vi "Attenuator Append Group Data Fields.vi"(10 "Attenuator Results":T1={"Measurement Cycles"=0, "Attenuator Test Parameters"={"Stimulus"={"ATT Stimulus"={"Normalize"=TRUE, "Value (dB)"=0.0}, "VNA Stimulus"={"Use Instrument Settings"=FALSE, "Blank Frequencies"=FALSE, "Sweep Type"=enum."Linear", "Sweep"={"Fstart"=500.0, "Fstop"=1500.0, "Units"=enum."MHz", "Points"=201}, "Power (dBm)"=999.0, "IFBW (Hz)"=-1.0, "Sweep Time (s)"=-1.0, "Calibration"={"State"=FALSE, "String"=""}}}, "Measurement"={"Step (dB)"=enum."0.25", "Start (dB)"=0.0, "Stop (dB)"=31.75}, "Limit"={"Maximum Error"=0.3}, "Normalization"={"Normalized?"=FALSE, "Normalization Values (dB)"=[]}}, "Measurement Values"={"# of Steps"=0, "Attenuation Variance"=[], "Frequency Sweeps"=[], "Peak Variance (dB)"=0.0, "Monotonic?"=FALSE}, "Pass?"=FALSE, "Instruments to Use"={"ATT Instrument Record"={"ixInstrument"=0, "sxInstrumentId"="", "sDriverId"="", "sDriverType"="", "sSerialNumber"="", "tLastCalibration"=timestamp(0 s since 1904-01-01), "tCalibrationDue"=timestamp(0 s since 1904-01-01), "sConfiguration"=""}, "VNA Instrument Record"={"ixInstrument"=0, "sxInstrumentId"="", "sDriverId"="", "sDriverType"="", "sSerialNumber"="", "tLastCalibration"=timestamp(0 s since 1904-01-01), "tCalibrationDue"=timestamp(0 s since 1904-01-01), "sConfiguration"=""}}} {"Attenuator Test Parameters"."Stimulus"."VNA Stimulus"."Sweep Time (s)" format="%.3g"}, 11 "Fields In":T13[](array[typedef])) -> (3 "Fields Out":T13[](array[typedef]))   [LabVIEW 2011]
uses:
  server/database/Fields/Field Record.ctl
  server/database/Fields/Field DataTypes.ctl
  server/database/Fields/Field NextItem.ctl
  TypeDefs/Attenuator Results.ctl
  TypeDefs/Attenuator Test Parameters.ctl
  TypeDefs/Attenuator Stimulus Parameters.ctl
  TypeDefs/Attenuator ATT Stimulus.ctl
  TypeDefs/Attenuator VNA Stimulus.ctl
  S Parameter/TypeDefs/SP Frequency Units.ctl
  TypeDefs/Attenuator VNA Calibration State.ctl
  TypeDefs/Attenuator Measurement Cluster.ctl
  TypeDefs/Attenuator Limit.ctl
  TypeDefs/Attenuator Calibration State.ctl
  TypeDefs/Attenuator Measurement Values.ctl
  server/database/Stations/Instruments/Instrument Record.ctl
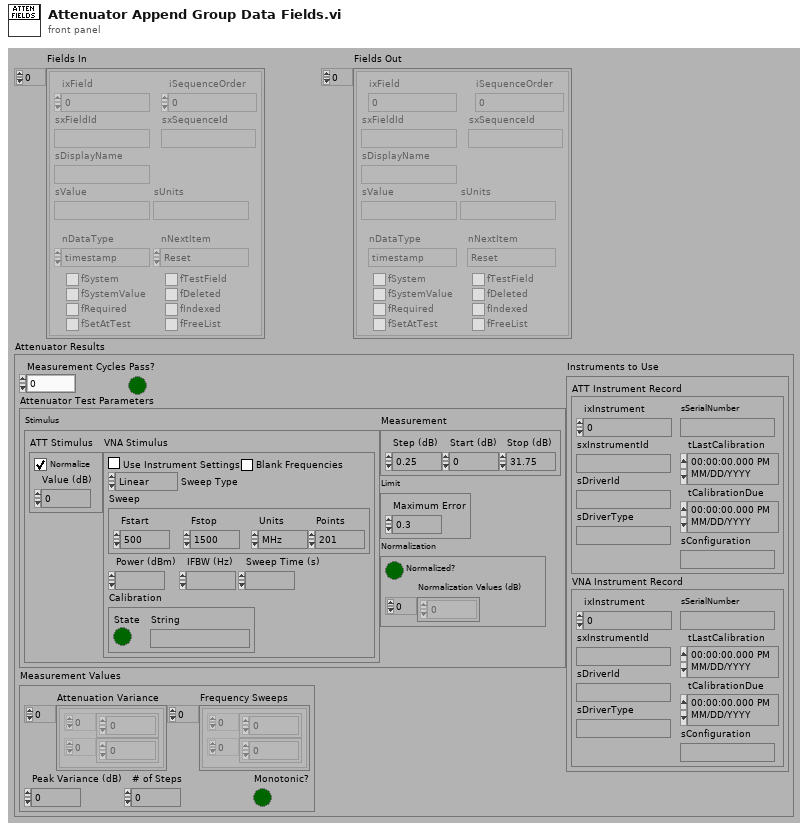
[diagram p1: front panel]
types:
  T1 = typedef "Attenuator Results.ctl" = cluster{"Measurement Cycles":i32, "Attenuator Test Parameters":T2, "Measurement Values":T11, "Pass?":bool, "Instruments to Use":cluster{"ATT Instrument Record":T12, "VNA Instrument Record":T12}}
  T2 = typedef "Attenuator Test Parameters.ctl" = cluster{"Stimulus":T3, "Measurement":T8, "Limit":T9, "Normalization":T10}
  T3 = typedef "Attenuator Stimulus Parameters.ctl" = cluster{"ATT Stimulus":T4, "VNA Stimulus":T5}
  T4 = typedef "Attenuator ATT Stimulus.ctl" = cluster{"Normalize":bool, "Value (dB)":dbl}
  T5 = typedef "Attenuator VNA Stimulus.ctl" = cluster{"Use Instrument Settings":bool, "Blank Frequencies":bool, "Sweep Type":enum32{"Linear", "Logarithmic", "List", "Power", "CW"}, "Sweep":cluster{"Fstart":dbl, "Fstop":dbl, "Units":T6, "Points":i32}, "Power (dBm)":dbl, "IFBW (Hz)":dbl, "Sweep Time (s)":dbl, "Calibration":T7}
  T6 = typedef "SP Frequency Units.ctl" = enum16{"Hz", "kHz", "MHz", "GHz", "Points"}
  T7 = typedef "Attenuator VNA Calibration State.ctl" = cluster{"State":bool, "String":string}
  T8 = typedef "Attenuator Measurement Cluster.ctl" = cluster{"Step (dB)":enum16{"0.25", "0.50", "1.00"}, "Start (dB)":dbl, "Stop (dB)":dbl}
  T9 = typedef "Attenuator Limit.ctl" = cluster{"Maximum Error":dbl}
  T10 = typedef "Attenuator Calibration State.ctl" = cluster{"Normalized?":bool, "Normalization Values (dB)":dbl[]}
  T11 = typedef "Attenuator Measurement Values.ctl" = cluster{"# of Steps":i32, "Attenuation Variance":cluster{"X":dbl[], "Y":dbl[]}[], "Frequency Sweeps":cluster{"X":dbl[], "Y":dbl[]}[], "Peak Variance (dB)":dbl, "Monotonic?":bool}
  T12 = typedef "Instrument Record.ctl" = cluster{"ixInstrument":i32, "sxInstrumentId":string, "sDriverId":string, "sDriverType":string, "sSerialNumber":string, "tLastCalibration":timestamp, "tCalibrationDue":timestamp, "sConfiguration":string}
  T13 = typedef "Field Record.ctl" = cluster{"ixField":i32, "iSequenceOrder":i32, "sxFieldId":string, "sxSequenceId":string, "sDisplayName":string, "sValue":string, "sUnits":string, "nDataType":T14, "nNextItem":T15, "fSystem":bool, "fSystemValue":bool, "fRequired":bool, "fSetAtTest":bool, "fTestField":bool, "fDeleted":bool, "fIndexed":bool, "fFreeList":bool}
  T14 = typedef "Field DataTypes.ctl" = enum32{"text", "numeric", "list", "timestamp", "boolean"}
  T15 = typedef "Field NextItem.ctl" = enum32{"Reset", "Retain", "Auto-Increment"}
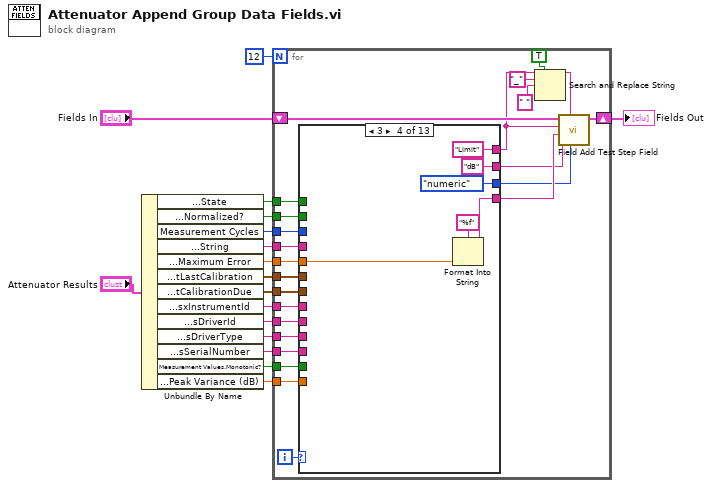
[diagram p0: block diagram]
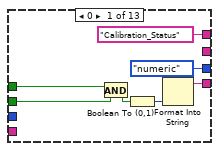
[diagram p2: hidden frame]
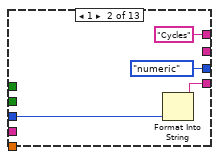
[diagram p3: hidden frame]
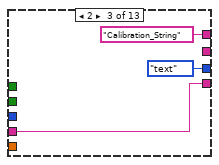
[diagram p4: hidden frame]
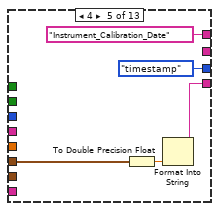
[diagram p5: hidden frame]
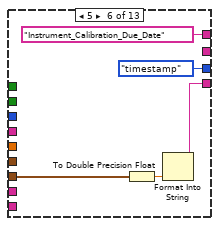
[diagram p6: hidden frame]
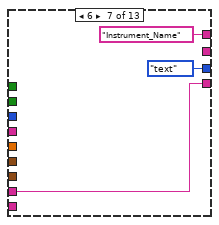
[diagram p7: hidden frame]
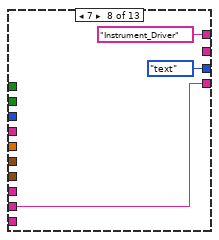
[diagram p8: hidden frame]
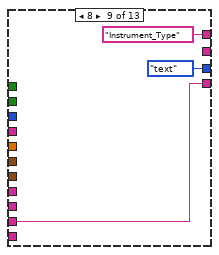
[diagram p9: hidden frame]
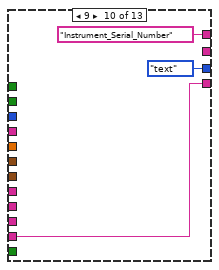
[diagram p10: hidden frame]
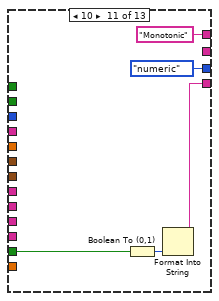
[diagram p11: hidden frame]
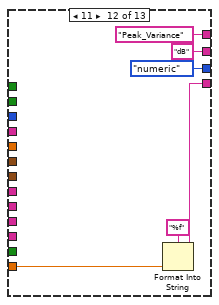
[diagram p12: hidden frame]
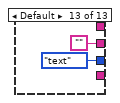
[diagram p13: hidden frame]
diagram:
  n1 = Unbundle By Name("Attenuator Results") -> ("Attenuator Test Parameters.Stimulus.VNA Stimulus.Calibration.State"=w3:bool, "Attenuator Test Parameters.Normalization.Normalized?"=w13:bool, "Measurement Cycles"=w12:i32, "Attenuator Test Parameters.Stimulus.VNA Stimulus.Calibration.String"=w11:string, "Attenuator Test Parameters.Limit.Maximum Error"=w10:dbl, "Instruments to Use.VNA Instrument Record.tLastCalibration"=w9:timestamp, "Instruments to Use.VNA Instrument Record.tCalibrationDue"=w4:timestamp, "Instruments to Use.VNA Instrument Record.sxInstrumentId"=w8:string, "Instruments to Use.ATT Instrument Record.sDriverId"=w7:string, "Instruments to Use.ATT Instrument Record.sDriverType"=w6:string, "Instruments to Use.ATT Instrument Record.sSerialNumber"=w5:string, "Measurement Values.Monotonic?"=w2:bool, "Measurement Values.Peak Variance (dB)"=w1:dbl)
  n2 = for {
    N: 12 -> [_]
    tunnel: w10 -> [w40]
    tunnel: w11 -> [w39]
    tunnel: w12 -> [w38]
    tunnel: w13 -> [w37]
    shift-right: [w35] -> w16
    shift-left: "Fields In" -> [w36]
    tunnel: w9 -> [w31]
    tunnel: w8 -> [w30]
    tunnel: w7 -> [w29]
    tunnel: w6 -> [w28]
    tunnel: w5 -> [w27]
    tunnel: w4 -> [w21]
    tunnel: w3 -> [w20]
    tunnel: w2 -> [w19]
    tunnel: w1 -> [w18]
    i -> [w41]
    n3 = case shown="3" w41 {
      tunnel: w40 -> [_ _ _ w58 _ _ _ _ _ _ _ _ _]
      tunnel: w39 -> [_ _ w53 _ _ _ _ _ _ _ _ _ _]
      tunnel: w38 -> [_ w50 _ _ _ _ _ _ _ _ _ _ _]
      tunnel: w37 -> [w44 _ _ _ _ _ _ _ _ _ _ _ _]
      tunnel: ["Calibration_Status" ("Field_ID") "Cycles" ("Field_ID") "Calibration_String" ("Field_ID") "Limit" ("Field_ID") "Instrument_Calibration_Date" ("Field_ID") "Instrument_Calibration_Due_Date" ("Field_ID") "Instrument_Name" ("Field_ID") "Instrument_Driver" ("Field_ID") "Instrument_Type" ("Field_ID") "Instrument_Serial_Number" ("Field_ID") "Monotonic" ("Field_ID") "Peak_Variance" ("Field_ID") _] -> w23
      tunnel: [Field_DataTypes."numeric" ("Data Type") Field_DataTypes."numeric" ("Data Type") Field_DataTypes."text" ("Data Type") Field_DataTypes."numeric" ("Data Type") Field_DataTypes."timestamp" ("Data Type") Field_DataTypes."timestamp" ("Data Type") Field_DataTypes."text" ("Data Type") Field_DataTypes."text" ("Data Type") Field_DataTypes."text" ("Data Type") Field_DataTypes."text" ("Data Type") Field_DataTypes."numeric" ("Data Type") Field_DataTypes."numeric" ("Data Type") Field_DataTypes."text" ("Data Type")] -> w33
      tunnel: [w47 w51 w53 w59 w63 w68 w72 w75 w78 w81 w84 w92 _] -> w34
      tunnel: [_ _ _ "dB" _ _ _ _ _ _ _ "dB" ""] -> w32
      tunnel: w31 -> [_ _ _ _ w62 _ _ _ _ _ _ _ _]
      tunnel: w30 -> [_ _ _ _ _ _ w72 _ _ _ _ _ _]
      tunnel: w29 -> [_ _ _ _ _ _ _ w75 _ _ _ _ _]
      tunnel: w28 -> [_ _ _ _ _ _ _ _ w78 _ _ _ _]
      tunnel: w27 -> [_ _ _ _ _ _ _ _ _ w81 _ _ _]
      tunnel: w21 -> [_ _ _ _ _ w67 _ _ _ _ _ _ _]
      tunnel: w20 -> [w43 _ _ _ _ _ _ _ _ _ _ _ _]
      tunnel: w19 -> [_ _ _ _ _ _ _ _ _ _ w85 _ _]
      tunnel: w18 -> [_ _ _ _ _ _ _ _ _ _ _ w90 _]
      frame 0 {
        n4 = And(x=w43, y=w44) -> (x .and. y?=w42:bool)
        n5 = Boolean To (0,1)(Boolean=w42) -> (0, 1=w45:i16)
        n6 = Format Into String(w45) -> (resulting string=w47:string)  [unwired: 3 in, 1 out]
      }
      frame 1 {
        n7 = Format Into String(w50) -> (resulting string=w51:string)  [unwired: 3 in, 1 out]
      }
      frame 2 {
      }
      frame 3 {
        n8 = Format Into String(format string="%f", w58) -> (resulting string=w59:string)  [unwired: 2 in, 1 out]
      }
      frame 4 {
        n9 = To Double Precision Float(number=w62) -> (double precision float=w64:dbl)
        n10 = Format Into String(w64) -> (resulting string=w63:string)  [unwired: 3 in, 1 out]
      }
      frame 5 {
        n11 = To Double Precision Float(number=w67) -> (double precision float=w69:dbl)
        n12 = Format Into String(w69) -> (resulting string=w68:string)  [unwired: 3 in, 1 out]
      }
      frame 6 {
      }
      frame 7 {
      }
      frame 8 {
      }
      frame 9 {
      }
      frame 10 {
        n13 = Boolean To (0,1)(Boolean=w85) -> (0, 1=w86:i16)
        n14 = Format Into String(w86) -> (resulting string=w84:string)  [unwired: 3 in, 1 out]
      }
      frame 11 {
        n15 = Format Into String(format string="%f", w90) -> (resulting string=w92:string)  [unwired: 2 in, 1 out]
      }
      frame Default {
      }
    }
    n16 = Search and Replace String(replace all?=TRUE ("replace all? (F)"), input string=w23, search string="_", replace string=" " ("replace string (\"\")")) -> (result string=w22:string)  [unwired: 1 in, 6 out]
    n17 = call "Field Add Test Step Field.vi"("nDataType"=w33, "sDisplayName"=w22, "sUnits"=w32, "sValue"=w34, "sxFieldId"=w23, "Fields In"=w36) -> ("Fields Out"=w35:T13[])  [unwired: 5 out]
  }
  "Fields Out" <- w16
